vi "meter global.vi"() -> ()   [LabVIEW 2016]
panel:
  in  "HIOKI  232 port":refnum<visa-resource-name>="COM3"
  in  "19073 485 port":refnum<visa-resource-name>="com21"
  in  "E4981 VISA resource name":refnum<visa-resource-name>="USB0::0x0957::0x0F09::MY48310636::INSTR"
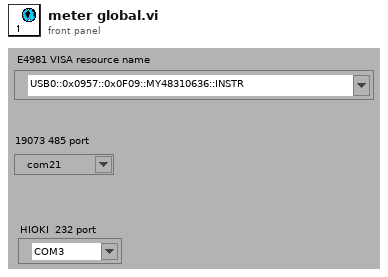
[diagram p1: front panel]
diagram:
